vi "(Incomplete) Gamma Function (obs).vi"(2 "a":dbl=nan format="%.2f", 3 "x":dbl format="%.2f") -> (1 "g(x, a)":dbl format="%.2f")   [LabVIEW 2014, in "NI_Gmath.lvlib"]
uses:
  NI_Gmath.lvlib
  Incomplete Gamma Function.vi
  Gamma Function.vi
panel:
  # "This VI is obsolete !!!\nYou should replace this VI in your diagram with the \n(Incomplete) Gamma Function VI.\n\nNOTE:   Please be aware that the new (Incomplete) Gamma\n             Function VI is a polymorphic VI. If you leave the a\n             input of this obsolete VI unwired, please use the \n             Gamma Function instance of the new (Incomplete)\n             Gamma Function VI."
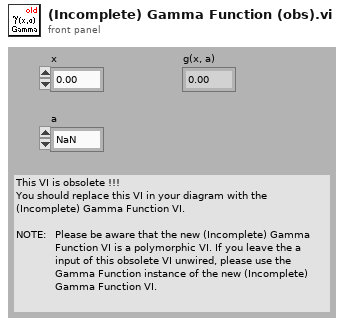
[diagram p1: front panel]
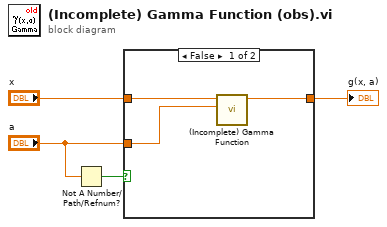
[diagram p0: block diagram]
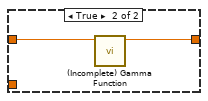
[diagram p2: hidden frame]
diagram:
  n1 = Not A Number/Path/Refnum?(number/path/refnum="a") -> (NaN/Path/Refnum?=w4:bool)
  n2 = case shown="False" w4 {
    tunnel: "x" -> [w7 w9]
    tunnel: [w5 w8] -> w1
    tunnel: "a" -> [w6 _]
    frame False {
      n3 = call-poly "(Incomplete) Gamma Function.vi"("a"=w6, "x"=w7) -> ("g(x, a)"=w5:dbl)  [unwired: 9 in]
    }
    frame True {
      n4 = call-poly "(Incomplete) Gamma Function.vi"("x"=w9) -> ("g(x)"=w8:dbl)  [unwired: 10 in]
    }
  }
  "g(x, a)" <- w1
